vi "VIQA Fix All.vi"(6 "Abort":refnum<vi>, 8 "error in (no error)":errorcluster, 9 "Slide":refnum<vi>, 10 "AuditMCLB":refnum<vi>, 11 "Project in":refnum<vi>) -> (0 "error out":errorcluster)   [LabVIEW 2018, in "VI Quality.lvlib"]
doc: "This VI fixes all VI properties and adds a disclaimer if not found."
uses:
  VI Quality.lvlib
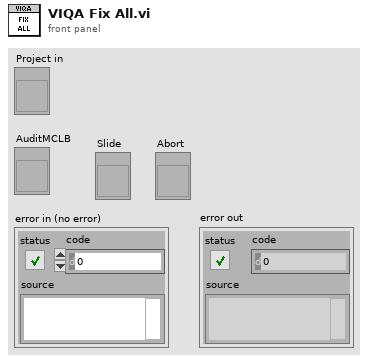
[diagram p1: front panel]
types:
  T1 = enum32{"invalid VI type", "Standard VI", "Control VI", "Global VI", "Polymorphic VI", "Configuration VI", "SubSystem", "Facade VI", "Method VI", "Statechart Diagram VI"}
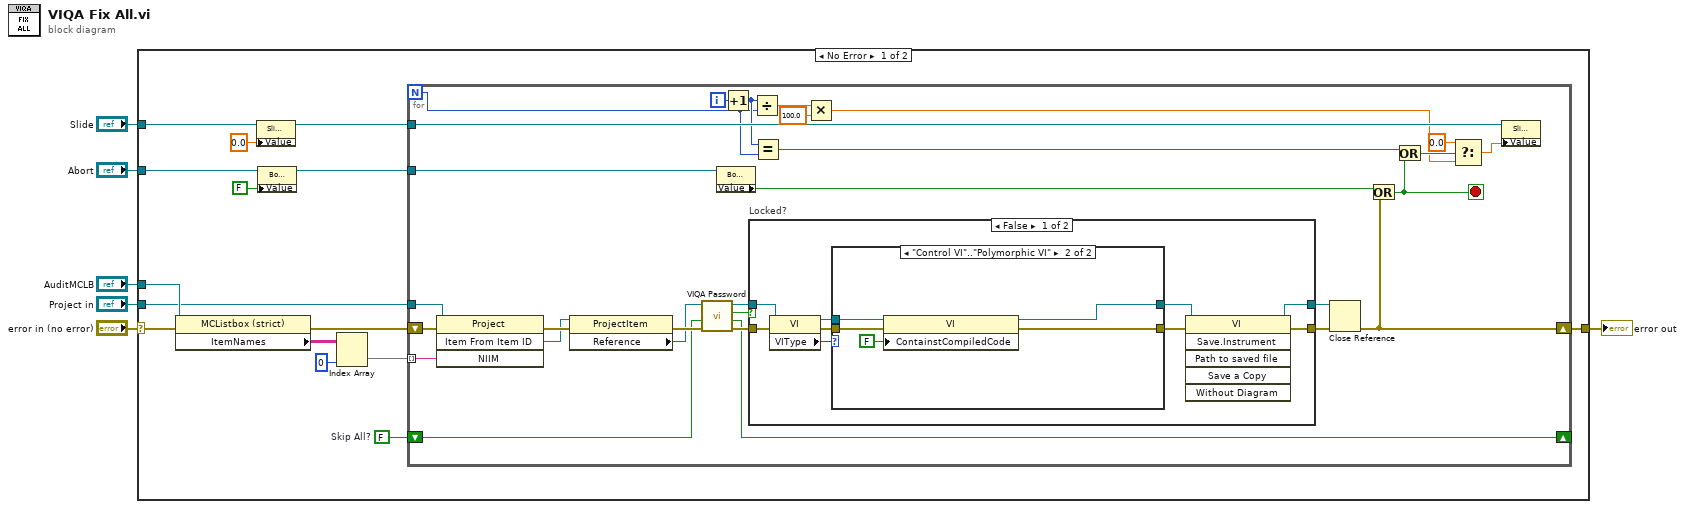
[diagram p0: block diagram]
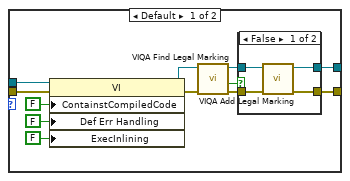
[diagram p2: hidden frame]
diagram:
  n1 = case shown="No Error" "error in (no error)" {
    selector: "error in (no error)" -> [w14 w85]
    tunnel: [w21 w85] -> w6
    tunnel: "AuditMCLB" -> [w17 _]
    tunnel: "Project in" -> [w15 _]
    tunnel: "Slide" -> [w13 _]
    tunnel: "Abort" -> [w10 _]
    frame No Error {
      w7 = FALSE  # Skip All?
      n2 = property class="MCListbox (strict)"(reference=w17, error in=w14) -> (error out=w16:errorcluster, "ItemNames"=w18:string[][])  [unwired: 1 out]
      n3 = property class="Slide (strict)"(reference=w13, "Value"=0.0) -> (reference out=w12:refnum<vi>)  [unwired: 1 in, 1 out]
      n4 = property class="Bool (strict)"(reference=w10, "Value"=FALSE) -> (reference out=w8:refnum<vi>)  [unwired: 1 in, 1 out]
      n5 = Index Array(array=w18, index (col)=0 ("disabled index (col)")) -> (element=w20:string[])  [unwired: 1 in]
      n6 = for {
        N -> [w45]
        tunnel: w15 -> [w32]
        tunnel: w20 -> [w31] mode=indexing
        shift-right: [w23] -> w21
        shift-left: w16 -> [w33]
        tunnel: w12 -> [w50]
        tunnel: w8 -> [w37]
        shift-right: [w24] -> _
        shift-left: w7 -> [w25]
        i -> [w49]
        stop <- w38 stop-if-true
        n7 = invoke class="Project" method="Item From Item ID"(reference=w32, error in=w33, "NIIM"=w31) -> (error out=w35:errorcluster, "GetItemFromNIIM"=w34:refnum<vi>)  [unwired: 1 in, 2 out]
        n8 = property class="ProjectItem"(reference=w34, error in=w35) -> (error out=w30:errorcluster, "Reference"=w29:refnum<vi>)  [unwired: 1 out]
        n9 = call "VIQA Password.vi"("error in (no error)"=w30, "Skip All? (F)"=w25, "VI Refnum"=w29) -> ("error out"=w27:errorcluster, "Skip All?"=w24:bool, "Locked"=w26:bool, "dup VI Refnum"=w28:refnum<vi>)  [unwired: 5 in]
        n10 = property class="Bool (strict)"(reference=w37) -> ("Value"=w36:bool)  [unwired: 1 in, 2 out]
        n11 = Increment(x=w49) -> (x+1=w46:i32)
        n12 = case "Locked?" shown="False" w26 {
          tunnel: w27 -> [w56 w84]
          tunnel: w28 -> [w55 w83]
          tunnel: [w53 w84] -> w39
          tunnel: [w51 w83] -> w22
          frame False {
            n13 = property class="VI"(reference=w55, error in=w56) -> (reference out=w57:refnum<vi>, error out=w59:errorcluster, "VIType"=w58:T1)
            n14 = case shown="\"Control VI\"..\"Polymorphic VI\"" w58 {
              tunnel: [w64 w82] -> w54
              tunnel: [w62 w81] -> w52
              tunnel: w59 -> [w71 w80]
              tunnel: w57 -> [w70 w79]
              frame Default {
                n15 = property class="VI"(reference=w70, error in=w71, "ContainstCompiledCode"=FALSE ("Contains Compiled Code"), "Def Err Handling"=FALSE ("Automatic Error Handling"), "ExecInlining"=FALSE ("Execution:Inline SubVI")) -> (reference out=w68:refnum<vi>, error out=w69:errorcluster)
                n16 = call "VIQA Find Legal Marking.vi"("error in (no error)"=w69, "VI Refnum"=w68) -> ("error out"=w65:errorcluster, "Found?"=w61:bool, "dup VI Refnum"=w63:refnum<vi>)  [unwired: 4 in, 3 out]
                n17 = case shown="False" w61 {
                  tunnel: w65 -> [w75 w76]
                  tunnel: [w74 w76] -> w64
                  tunnel: w63 -> [w73 w77]
                  tunnel: [w72 w77] -> w62
                  frame False {
                    n18 = call "VIQA Add Legal Marking.vi"("error in (no error)"=w75, "VI Refnum"=w73) -> ("error out"=w74:errorcluster, "dup VI Refnum"=w72:refnum<vi>)  [unwired: 8 in]
                  }
                  frame True {
                  }
                }
              }
              frame "Control VI".."Polymorphic VI" {
                n19 = property class="VI"(reference=w79, error in=w80, "ContainstCompiledCode"=FALSE ("Contains Compiled Code")) -> (reference out=w81:refnum<vi>, error out=w82:errorcluster)
              }
            }
            n20 = invoke class="VI" method="Save.Instrument"(reference=w52, error in=w54) -> (reference out=w51:refnum<vi>, error out=w53:errorcluster)  [unwired: 4 in, 4 out]
          }
          frame True {
          }
        }
        n21 = Divide(x=w46, y=w45) -> (x/y=w48:dbl)
        n22 = Equal?(x=w46, y=w45) -> (x = y?=w44:bool)
        n23 = Multiply(x=w48, y=100.0) -> (x*y=w42:dbl)
        n24 = Close Reference(reference=w22, error in (no error)=w39) -> (error out=w23:errorcluster)
        n25 = Or(x=w36, y=w23) -> (x .or. y?=w38:bool)
        n26 = Or(x=w44, y=w38) -> (x .or. y?=w43:bool)
        n27 = Select(t=0.0, s=w43, f=w42) -> (s? t:f=w40:dbl)
        n28 = property class="Slide (strict)"(reference=w50, "Value"=w40) -> ()  [unwired: 1 in, 2 out]
      }
    }
    frame Error {
    }
  }
  "error out" <- w6
